vi "better extinction.vi"(8 "standard cluster":T1={"Description"="", "Setup"={"integration time"=0.5, "rinse time"=10.0, "sample time"=10.0, "sample type"=0}, "Concentrations"=[], "Absorbance"=[], "Analyst"="", "Concentration units"="", "Good"=[]} {"Absorbance" format="%.2e"; "Concentrations" format="%.3e"; "Setup"."sample type" items=["Sample Cuvet", "Sipper Cell", "No Dialog"]; "Setup"."sample time" min=0.0 max=100.0 step=1.0 format="%.1f"; "Setup"."rinse time" min=0.0 max=100.0 step=1.0 format="%.1f"; "Setup"."integration time" format="%.1f"}, 11 "Cest":dbl format="%.2e") -> (2 "good":bool[](array[boolean]), 3 "extinction":dbl[](array[numeric]) format="%.2f")   [LabVIEW 2015]
uses:
  standard cluster.ctl
  settings.ctl
panel:
  out "floor(x/y)":dbl format="%.2f"
  out "x-y*floor(x/y)":dbl format="%.2f"
  out "interpolation":T3(ring)
  out "fractional index or x":dbl format="%.2f"
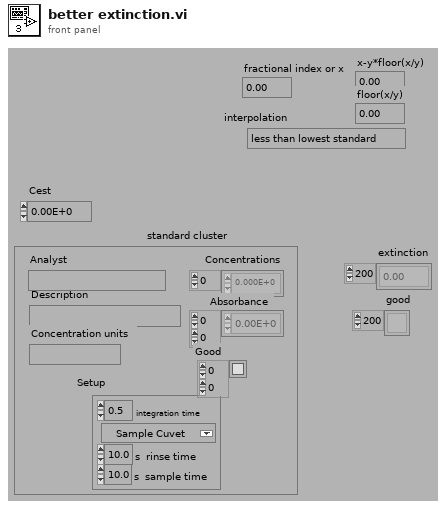
[diagram p1: front panel]
types:
  T1 = typedef "standard cluster.ctl" = cluster{"Description":string, "Setup":T2, "Concentrations":dbl[], "Absorbance":dbl[][], "Analyst":string, "Concentration units":string, "Good":bool[][]}
  T2 = typedef "settings.ctl" = cluster{"integration time":sgl, "rinse time":dbl[unit], "sample time":dbl[unit], "sample type":u16}
  T3 = enum16{"less than lowest standard", "interpolate", "greater than highest standard"}
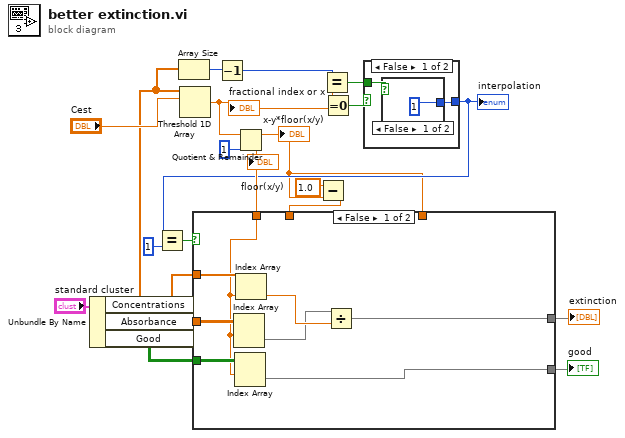
[diagram p0: block diagram]
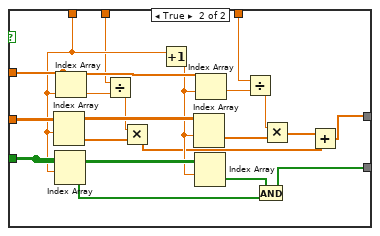
[diagram p2: hidden frame]
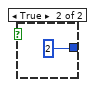
[diagram p3: hidden frame]
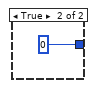
[diagram p4: hidden frame]
diagram:
  n1 = Unbundle By Name("standard cluster") -> ("Concentrations"=w14:dbl[], "Absorbance"=w10:dbl[][], "Good"=w9:bool[][])
  n2 = Array Size(array=w14) -> (size(s)=w19:i32)
  n3 = Threshold 1D Array(2:"Cest", 3:w14) -> (0:w13:dbl)  [unwired: 1 in]
  "fractional index or x" <- w13
  n4 = Decrement(x=w19) -> (x-1=w18:i32)
  n5 = Quotient & Remainder(x=w13, y=1) -> (x-y*floor(x/y)=w1:dbl, floor(x/y)=w11:dbl)
  "x-y*floor(x/y)" <- w1
  "floor(x/y)" <- w11
  n6 = Subtract(x=1.0, y=w1) -> (x-y=w2:dbl)
  n7 = Equal?(x=w18, y=w13) -> (x = y?=w16:bool)
  n8 = Equal To 0?(x=w13) -> (x = 0?=w17:bool)
  n9 = case shown="False" w17 {
    tunnel: [w21 0] -> w7
    tunnel: w16 -> [w22 _]
    frame False {
      n10 = case shown="False" w22 {
        tunnel: [1 2] -> w21
        frame False {
        }
        frame True {
        }
      }
    }
    frame True {
    }
  }
  "interpolation" <- w7
  n11 = Equal?(x=w7, y=1) -> (x = y?=w5:bool)
  n12 = case shown="False" w5 {
    tunnel: w14 -> [w33 w52]
    tunnel: w10 -> [w31 w51]
    tunnel: w9 -> [w29 w50]
    tunnel: [w28 w37] -> w4
    tunnel: [w27 w34] -> w3
    tunnel: w11 -> [w26 w49]
    tunnel: w2 -> [_ w46]
    tunnel: w1 -> [_ w43]
    frame False {
      n13 = Index Array(array=w31, index (row)=w26) -> (element=w30:dbl[])  [unwired: 1 in]
      n14 = Index Array(array=w29, index (row)=w26) -> (element=w27:bool[])  [unwired: 1 in]
      n15 = Index Array(array=w33, index=w26) -> (element=w32:dbl)
      n16 = Divide(x=w30, y=w32) -> (x/y=w28:dbl[])
    }
    frame True {
      n17 = Index Array(array=w51, index (row)=w49) -> (element=w44:dbl[])  [unwired: 1 in]
      n18 = Index Array(array=w50, index (row)=w49) -> (element=w35:bool[])  [unwired: 1 in]
      n19 = Index Array(array=w52, index=w49) -> (element=w47:dbl)
      n20 = Divide(x=w46, y=w47) -> (x/y=w45:dbl)
      n21 = Multiply(x=w45, y=w44) -> (x*y=w39:dbl[])
      n22 = Increment(x=w49) -> (x+1=w48:dbl)
      n23 = Index Array(array=w51, index (row)=w48) -> (element=w40:dbl[])  [unwired: 1 in]
      n24 = Index Array(array=w50, index (row)=w48) -> (element=w36:bool[])  [unwired: 1 in]
      n25 = Index Array(array=w52, index=w48) -> (element=w42:dbl)
      n26 = Divide(x=w43, y=w42) -> (x/y=w41:dbl)
      n27 = And(x=w36, y=w35) -> (x .and. y?=w34:bool[])
      n28 = Multiply(x=w41, y=w40) -> (x*y=w38:dbl[])
      n29 = Add(x=w38, y=w39) -> (x+y=w37:dbl[])
    }
  }
  "good" <- w3
  "extinction" <- w4
